vi "Y_switch_heating.vi"(9 "Y":T4={"Y_HSw"=1, "Y_HSetState"=enum."auto", "Y_ASetState"=enum."auto", "Y_DSetState"=enum."auto"}, 10 "Z":cluster{"Z_State":T1, "ZM_State":T2}={"Z_State"=enum."disabled", "ZM_State"=enum."stop"}, 11 "Y_LSw (2-auto)":u32=2) -> (2 "Y_SetState":T3=enum."auto", 3 "Y_Source":T5=enum."local disabled")   [LabVIEW 2019, in "Heating.lvlib"]
doc: "Y_Source – источник выхода\n 0 – initialize (Инициализация)\n 1 – local disabled (Выведен из работы по месту)\n 2 – local hand (Ручной местный)\n 3 – hand (Ручной контроллера)\n 4 – auto (Автомат контроллера)\n 5 – dist (Дистанционный)\nY_SetState заданное состояние выхода:\n 0 – initialize (Инициализация) \n 1 – alarm (Аварийное значение)\n 2 – min (Минимальное значение)\n 3 – stop (Остановлен)\n 4 – forced (Принудительное (ручное) задание)\n 5 – auto (Автомат (ПИД регулятор))\n 6 – max (Максимум)"
uses:
  Heating.lvlib
  ctl/Y_source.ctl
  ctl/Y_state.ctl
  ctl/Z_State.ctl
  ctl/ZM_State.ctl
panel:
  # "Входы\nY_LSw – переключатель р/а. 1 приоритет\n     0 – откл\n     1 – ручной (местный)\n     2 – автомат\nY_HSw – источник выхода из меню. 2 приоритет\n     0 – ручной контроллера\n     1 – автомат контроллера\n     2 – дистационный\nY_HSetState – заданное состояние в меню или на панели\nY_ASetState – автоматически заданное состояние от вышестоящего алгоритма\nY_DSetState – дистанционно заданное состояние\n     ..0 – initialize (Инициализация)  -> 4 – автомат \n     1 – alarm (Аварийное значение)\n     2 – min (Минимальное значение)\n     3 – stop (Остановлен)\n     4 – forced (Принудительное (ручное) задание)\n     5 – auto (Автомат (ПИД регулятор))\n     6 – max (Максимум)\n     7.. -> 4 – автомат"
  # "Выходы\nY_Source – источник выхода\n     0 – initialize (Инициализация)\n     1 – local disabled (Выведен из работы по месту)\n     2 – local hand (Ручной местный)\n     3 – hand (Ручной контроллера)\n     4 – auto (Автомат контроллера)\n     5 – dist (Дистанционный)\nY_SetState заданное состояние выхода:\n     0 – initialize (Инициализация) \n     1 – alarm (Аварийное значение)\n     2 – min (Минимальное значение)\n     3 – stop (Остановлен)\n     4 – forced (Принудительное (ручное) задание)\n     5 – auto (Автомат (ПИД регулятор))\n     6 – max (Максимум)"
  # "Z_State(Z3) состояние автомата механизма:\n     1 – alarm (авария)\n     2 – disabled (выведен из работы)\n     3 – not ready (не готов к работе)\n     4 – stop (стоп - готов к работе)\n     5 – reserv (резерв)\n     6 – switched off (отключается)\n     8 – switched on (включается)\n     9 – check (проверка работоспособности)\n     10 – on min (включен на минимуме)\n     11 – increase out (увеличение рабочего параметра)\n     12 – on (включен)\n     13 – decrease out (уменьшение рабочего параметра)\n     14 – on max (включен на максимуме)\nZM_State Состояние нагревателя и пусковой аппаратуры\n     0 – инициализация\n     1 – остановлен\n     2 – получен сигнал на пуск\n     3 – подан сигнал на включение контактора\n     4 – контактор включен, разогрев\n     5 – нагреватель включен\n     6 – получен сигнал на останов нагревателя (задержка перед отключением)\n     7 – снижение нагрузки\n     8 – снят сигнал на пуск контактора\n     9 – контактор отключен, охлаждение\n     10 – задержка повторного старта"
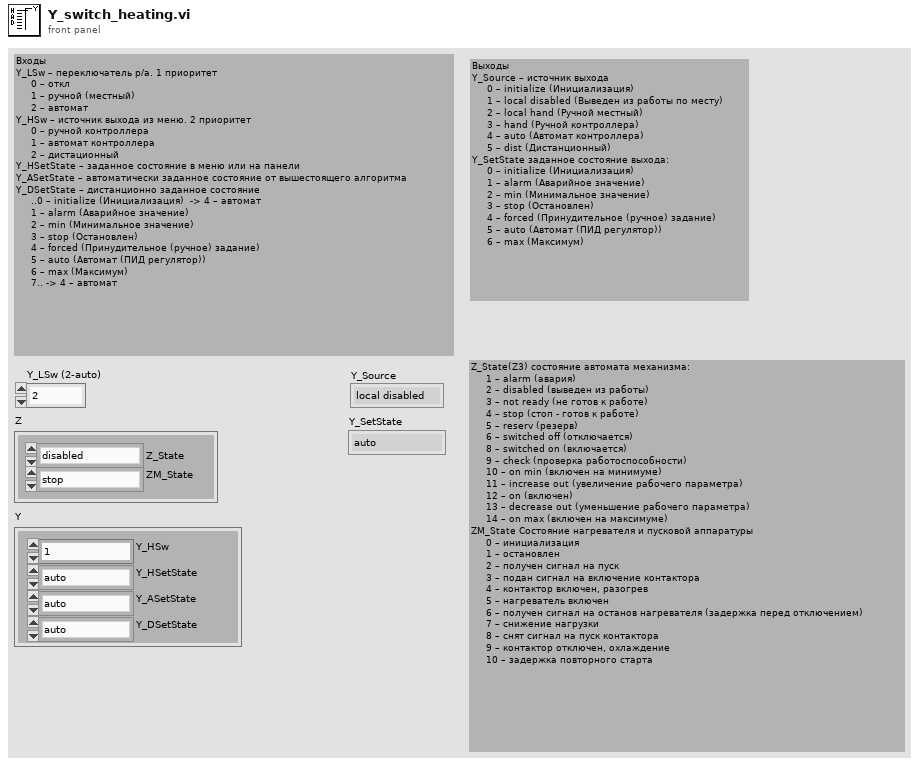
[diagram p1: front panel]
types:
  T1 = typedef "Heating.lvlib/Z_State.ctl" = enum8{"initialization", "alarm", "disabled", "not ready", "stop ready", "reserv", "switched off", "reserv2", "switched on", "check", "on min", "decrease out", "on", "increase out", "on max"}
  T2 = typedef "Heating.lvlib/ZM_State.ctl" = enum8{"initialization", "stop", "start_cmd", "contactor_on_cmd", "heating", "on", "stop_cmd", "power_down", "contactor_off_cmd", "cooling", "restart_delay"}
  T3 = typedef "Heating.lvlib/Y_state.ctl" = enum8{"initialize", "alarm", "min", "stop", "hand", "auto", "max"}
  T4 = cluster{"Y_HSw":u32, "Y_HSetState":T3, "Y_ASetState":T3, "Y_DSetState":T3}
  T5 = typedef "Heating.lvlib/Y_source.ctl" = enum8{"initialize", "local disabled", "local hand", "hand", "auto", "dist"}
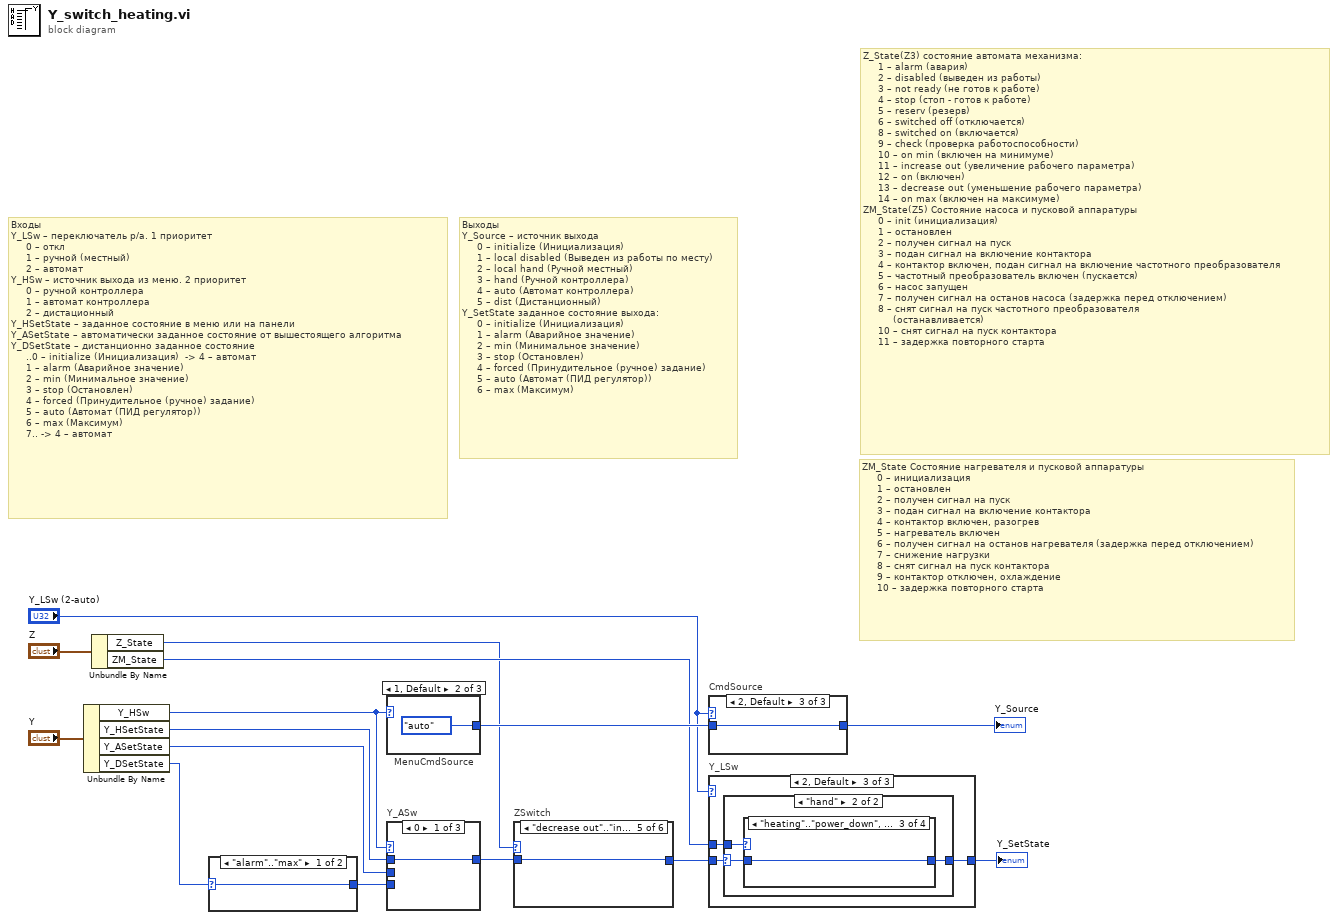
[diagram p0: block diagram]
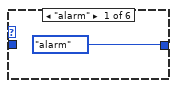
[diagram p2: hidden frame]
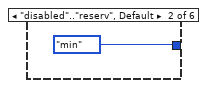
[diagram p3: hidden frame]
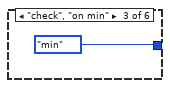
[diagram p4: hidden frame]
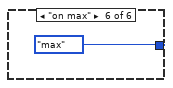
[diagram p6: hidden frame]
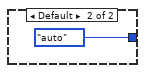
[diagram p7: hidden frame]
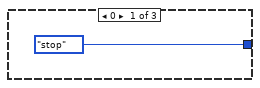
[diagram p10: hidden frame]
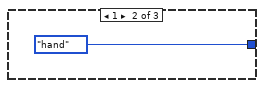
[diagram p11: hidden frame]
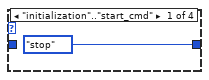
[diagram p13: hidden frame]
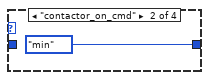
[diagram p14: hidden frame]
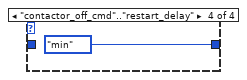
[diagram p15: hidden frame]
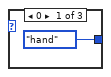
[diagram p16: hidden frame]
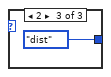
[diagram p17: hidden frame]
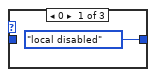
[diagram p18: hidden frame]
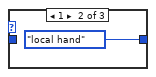
[diagram p19: hidden frame]
diagram:
  # "ZM_State Состояние нагревателя и пусковой аппаратуры\n     0 – инициализация\n     1 – остановлен\n     2 – получен сигнал на пуск\n     3 – подан сигнал на включение контактора\n     4 – контактор включен, разогрев\n     5 – нагреватель включен\n     6 – получен сигнал на останов нагревателя (задержка перед отключением)\n     7 – снижение нагрузки\n     8 – снят сигнал на пуск контактора\n     9 – контактор отключен, охлаждение\n     10 – задержка повторного старта"
  # "Z_State(Z3) состояние автомата механизма:\n     1 – alarm (авария)\n     2 – disabled (выведен из работы)\n     3 – not ready (не готов к работе)\n     4 – stop (стоп - готов к работе)\n     5 – reserv (резерв)\n     6 – switched off (отключается)\n     8 – switched on (включается)\n     9 – check (проверка работоспособности)\n     10 – on min (включен на минимуме)\n     11 – increase out (увеличение рабочего параметра)\n     12 – on (включен)\n     13 – decrease out (уменьшение рабочего параметра)\n     14 – on max (включен на максимуме)\nZM_State(Z5) Состояние насоса и пусковой аппаратуры\n     0 – init (инициализация)\n     1 – остановлен\n     2 – получен сигнал на пуск\n     3 – подан сигнал на включение контактора\n     4 – контактор включен, подан сигнал на включение частотного преобразователя\n     5 – частотный преобразователь включен (пускается)\n     6 – насос запущен\n     7 – получен сигнал на останов насоса (задержка перед отключением)\n     8 – снят сигнал на пуск частотного преобразователя\n          (останавливается)\n     10 – снят сигнал на пуск контактора\n     11 – задержка повторного старта"
  # "Входы\nY_LSw – переключатель р/а. 1 приоритет\n     0 – откл\n     1 – ручной (местный)\n     2 – автомат\nY_HSw – источник выхода из меню. 2 приоритет\n     0 – ручной контроллера\n     1 – автомат контроллера\n     2 – дистационный\nY_HSetState – заданное состояние в меню или на панели\nY_ASetState – автоматически заданное состояние от вышестоящего алгоритма\nY_DSetState – дистанционно заданное состояние\n     ..0 – initialize (Инициализация)  -> 4 – автомат \n     1 – alarm (Аварийное значение)\n     2 – min (Минимальное значение)\n     3 – stop (Остановлен)\n     4 – forced (Принудительное (ручное) задание)\n     5 – auto (Автомат (ПИД регулятор))\n     6 – max (Максимум)\n     7.. -> 4 – автомат"
  # "Выходы\nY_Source – источник выхода\n     0 – initialize (Инициализация)\n     1 – local disabled (Выведен из работы по месту)\n     2 – local hand (Ручной местный)\n     3 – hand (Ручной контроллера)\n     4 – auto (Автомат контроллера)\n     5 – dist (Дистанционный)\nY_SetState заданное состояние выхода:\n     0 – initialize (Инициализация) \n     1 – alarm (Аварийное значение)\n     2 – min (Минимальное значение)\n     3 – stop (Остановлен)\n     4 – forced (Принудительное (ручное) задание)\n     5 – auto (Автомат (ПИД регулятор))\n     6 – max (Максимум)"
  n1 = Unbundle By Name("Y") -> ("Y_HSw"=w7:u32, "Y_HSetState"=w6:T3, "Y_ASetState"=w5:T3, "Y_DSetState"=w4:T3)
  n2 = Unbundle By Name("Z") -> ("Z_State"=w1:T1, "ZM_State"=w2:T2)
  n3 = case shown="\"alarm\"..\"max\"" w4 {
    selector: w4 -> [w16 _]
    tunnel: [w16 Y_state."auto" ("X1(SetState)")] -> w13
    frame "alarm".."max" {
    }
    frame Default {
    }
  }
  n4 = case "MenuCmdSource" shown="1, Default" w7 {
    tunnel: [Y_source."hand" ("Z1(CmdSource) 3") Y_source."auto" ("Z1(CmdSource) 3") Y_source."dist" ("Z1(CmdSource) 3")] -> w15
    frame 0 {
    }
    frame 1, Default {
    }
    frame 2 {
    }
  }
  n5 = case "Y_ASw" shown="0" w7 {
    tunnel: [w21 w22 w23] -> w10
    tunnel: w6 -> [w21 _ _]
    tunnel: w13 -> [_ _ w23]
    tunnel: w5 -> [_ w22 _]
    frame 0 {
    }
    frame 1, Default {
    }
    frame 2 {
    }
  }
  n6 = case "ZSwitch" shown="\"decrease out\"..\"increase out\"" w1 {
    tunnel: [Y_state."alarm" ("Y_HSetState") Y_state."min" ("Y_HSetState") Y_state."min" ("Y_HSetState") w27 w28 Y_state."max" ("Y_HSetState")] -> w9
    tunnel: w10 -> [_ _ _ w27 w28 _]
    frame "alarm" {
    }
    frame "disabled".."reserv", Default {
    }
    frame "check", "on min" {
    }
    frame "switched off", "switched on" {
    }
    frame "decrease out".."increase out" {
    }
    frame "on max" {
    }
  }
  n7 = case "CmdSource" shown="2, Default" "Y_LSw (2-auto)" {
    tunnel: [Y_source."local disabled" ("Z1(CmdSource) 3") Y_source."local hand" ("Z1(CmdSource) 3") w32] -> w12
    tunnel: w15 -> [_ _ w32]
    frame 0 {
    }
    frame 1 {
    }
    frame 2, Default {
    }
  }
  "Y_Source" <- w12
  n8 = case "Y_LSw" shown="2, Default" "Y_LSw (2-auto)" {
    tunnel: [Y_state."stop" ("X1(SetState)") Y_state."hand" ("X1(SetState)") w36] -> w11
    tunnel: w9 -> [_ _ w37]
    tunnel: w2 -> [_ _ w35]
    frame 0 {
    }
    frame 1 {
    }
    frame 2, Default {
      n9 = case shown="\"hand\"" w37 {
        selector: w37 -> [w38 w41]
        tunnel: [w38 w40] -> w36
        tunnel: w35 -> [_ w39]
        frame "initialize", Default {
        }
        frame "hand" {
          n10 = case shown="\"heating\"..\"power_down\", Default" w39 {
            tunnel: w41 -> [_ _ w44 _]
            tunnel: [Y_state."stop" ("Y_HSetState") Y_state."min" ("Y_HSetState") w44 Y_state."min" ("Y_HSetState")] -> w40
            frame "initialization".."start_cmd" {
            }
            frame "contactor_on_cmd" {
            }
            frame "heating".."power_down", Default {
            }
            frame "contactor_off_cmd".."restart_delay" {
            }
          }
        }
      }
    }
  }
  "Y_SetState" <- w11
